vi "CRYFind Insert Locaction in Tree.vi"(6 "sData In":string[](array[string]), 7 "sAction":string, 8 "Index in Step":i32, 9 "Index in Tree":i32, 10 "ParentTag In":string, 11 "Tree in":refnum<vi>) -> (1 "ChildIndex":i32, 2 "ParentTag Out":string, 3 "Tree Out":refnum<vi>)   [LabVIEW 2013]
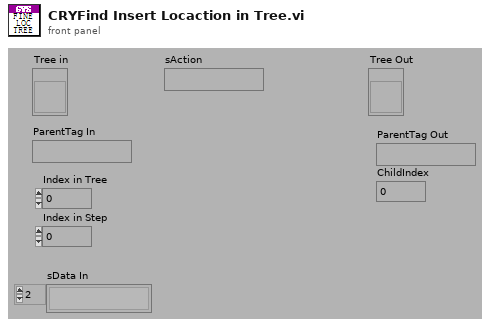
[diagram p1: front panel]
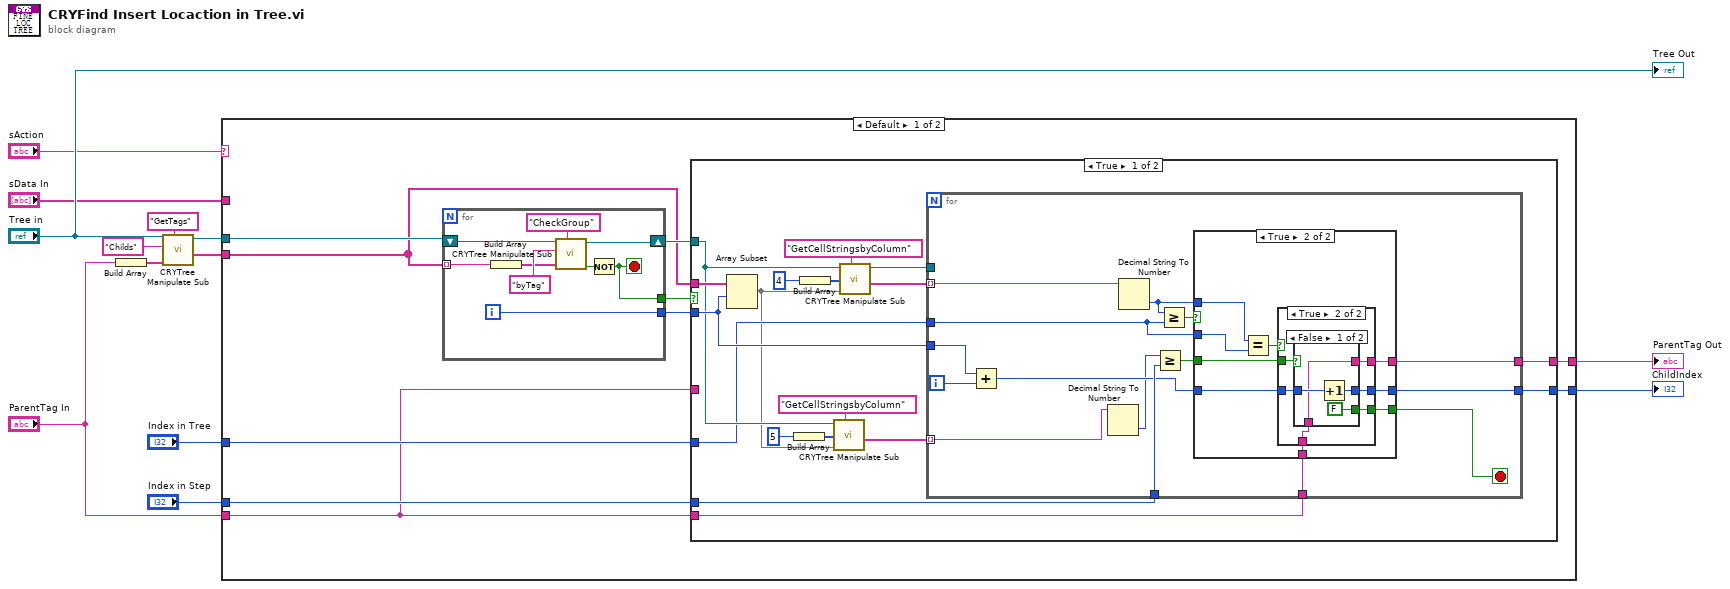
[diagram p0: block diagram]
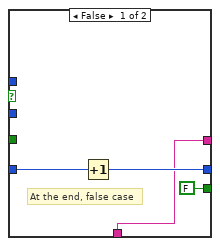
[diagram p2: hidden frame]
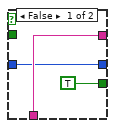
[diagram p3: hidden frame]
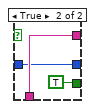
[diagram p4: hidden frame]
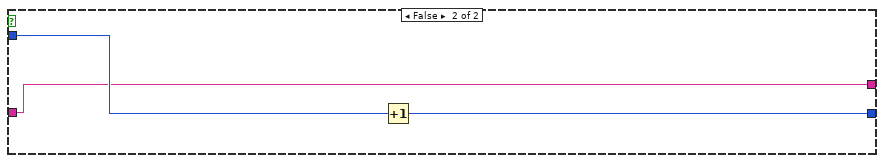
[diagram p5: hidden frame]
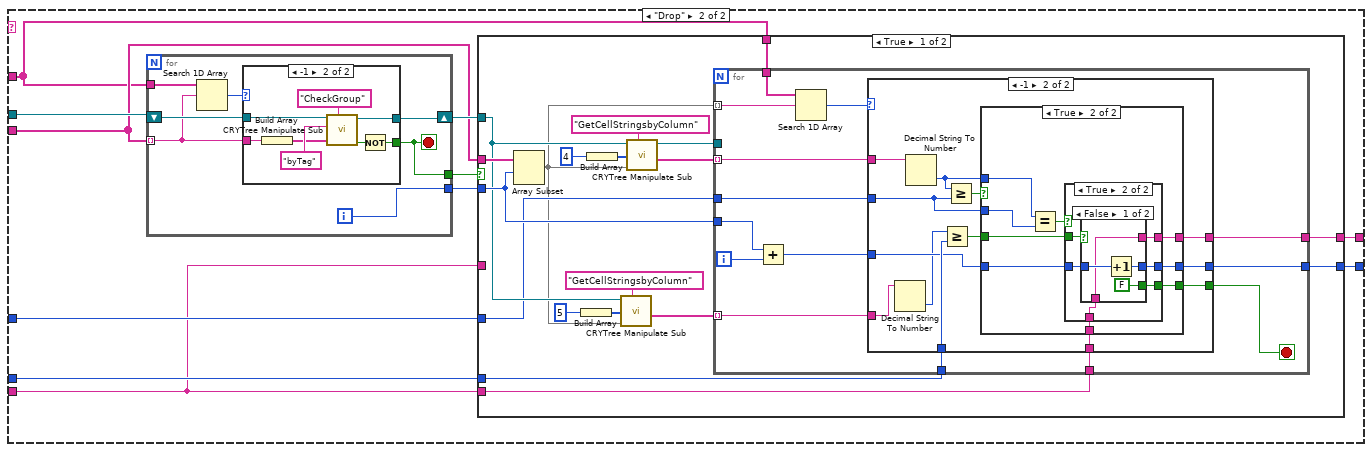
[diagram p6: hidden frame]
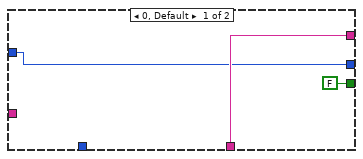
[diagram p7: hidden frame]
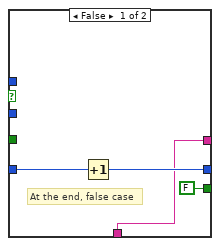
[diagram p8: hidden frame]
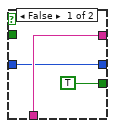
[diagram p9: hidden frame]
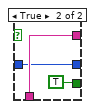
[diagram p10: hidden frame]
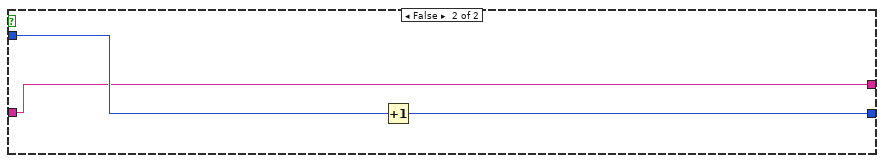
[diagram p11: hidden frame]
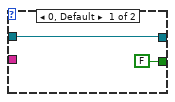
[diagram p12: hidden frame]
diagram:
  n1 = Build Array("ParentTag In") -> (w11:string[])
  n2 = call "CRYTree Manipulate Sub.vi"("sAction"="GetTags", "sData"=w11, "sOption"="Childs", "Tree in"="Tree in") -> ("sData Out"=w3:string[], "Tree Out"=w10:refnum<vi>)  [unwired: 3 in, 3 out]
  n3 = case shown="Default" "sAction" {
    tunnel: w10 -> [w23 w108]
    tunnel: [w19 w104] -> w8
    tunnel: [w18 w103] -> w7
    tunnel: "Index in Tree" -> [w17 w102]
    tunnel: "Index in Step" -> [w16 w101]
    tunnel: "ParentTag In" -> [w15 w100]
    tunnel: w3 -> [w14 w99]
    tunnel: "sData In" -> [_ w98]
    frame Default {
      n4 = for {
        tunnel: w14 -> [w90] mode=indexing
        tunnel: [w95] -> w21
        shift-right: [w91] -> w22
        shift-left: w23 -> [w93]
        tunnel: [w89] -> w20
        i -> [w95]
        stop <- w89 stop-if-true
        n5 = Build Array(w90) -> (w92:string[])
        n6 = call "CRYTree Manipulate Sub.vi"("sAction"="CheckGroup", "sData"=w92, "sOption"="byTag", "Tree in"=w93) -> ("bData out"=w96:bool, "Tree Out"=w91:refnum<vi>)  [unwired: 3 in, 3 out]
        n7 = Not(x=w96) -> (.not. x?=w89:bool)
      }
      n8 = case shown="True" w20 {
        tunnel: w22 -> [w32 _]
        tunnel: [w27 w87] -> w19
        tunnel: [w26 w86] -> w18
        tunnel: w14 -> [w37 _]
        tunnel: w21 -> [w36 w88]
        tunnel: w17 -> [w30 _]
        tunnel: w16 -> [w29 _]
        tunnel: w15 -> [w28 _]
        tunnel: w15 -> [_ w87]
        frame True {
          n9 = Array Subset(array=w37, index=w36) -> (w25:string[])  [unwired: 1 in]
          n10 = Build Array(5 ("nData 2")) -> (w35:i32[])
          n11 = Build Array(4 ("nData 2")) -> (w39:i32[])
          n12 = call "CRYTree Manipulate Sub.vi"("sAction"="GetCellStringsbyColumn", "sData"=w25, "nData"=w35, "Tree in"=w32) -> ("sData Out"=w31:string[])  [unwired: 3 in, 4 out]
          n13 = call "CRYTree Manipulate Sub.vi"("sAction"="GetCellStringsbyColumn", "sData"=w25, "nData"=w39, "Tree in"=w32) -> ("sData Out"=w38:string[], "Tree Out"=w24:refnum<vi>)  [unwired: 3 in, 3 out]
          n14 = for {
            tunnel: w38 -> [w56] mode=indexing
            tunnel: w30 -> [w47]
            tunnel: w36 -> [w54]
            tunnel: w31 -> [w53] mode=indexing
            tunnel: w29 -> [w52]
            tunnel: w28 -> [w51]
            tunnel: [w49] -> w27
            tunnel: [w48] -> w26
            tunnel: w24 -> [_]
            i -> [w55]
            stop <- w46 stop-if-true
            n15 = Add(x=w54, y=w55) -> (x+y=w50:i32)
            n16 = Decimal String To Number(string=w53) -> (number=w45:i32)  [unwired: 2 in, 1 out]
            n17 = Decimal String To Number(string=w56) -> (number=w42:i32)  [unwired: 2 in, 1 out]
            n18 = Greater Or Equal?(x=w45, y=w52) -> (x >= y?=w43:bool)
            n19 = Greater Or Equal?(x=w42, y=w47) -> (x >= y?=w44:bool)
            n20 = case shown="True" w44 {
              tunnel: w51 -> [w57 w68]
              tunnel: w50 -> [w60 w65]
              tunnel: [w57 w67] -> w49
              tunnel: [w58 w66] -> w48
              tunnel: w47 -> [_ w62]
              tunnel: w43 -> [_ w64]
              tunnel: [FALSE w63] -> w46
              tunnel: w42 -> [_ w61]
              frame False {
                # "At the end, false case"
                n21 = Increment(x=w60) -> (x+1=w58:i32)
              }
              frame True {
                n22 = Equal?(x=w61, y=w62) -> (x = y?=w69:bool)
                n23 = case shown="True" w69 {
                  tunnel: w68 -> [w72 w76]
                  tunnel: [w72 w77] -> w67
                  tunnel: [w71 w75] -> w66
                  tunnel: w65 -> [w71 w74]
                  tunnel: w64 -> [_ w78]
                  tunnel: [TRUE w73] -> w63
                  frame False {
                  }
                  frame True {
                    n24 = case shown="False" w78 {
                      tunnel: [w79 w85] -> w77
                      tunnel: w76 -> [w79 w85]
                      tunnel: [w80 w84] -> w75
                      tunnel: w74 -> [w81 w84]
                      tunnel: [FALSE TRUE] -> w73
                      frame False {
                        n25 = Increment(x=w81) -> (x+1=w80:i32)
                      }
                      frame True {
                      }
                    }
                  }
                }
              }
            }
          }
        }
        frame False {
          n26 = Increment(x=w88) -> (x+1=w86:i32)
        }
      }
    }
    frame "Drop" {
      n27 = for {
        tunnel: w99 -> [w190] mode=indexing
        tunnel: [w196] -> w106
        shift-right: [w194] -> w107
        shift-left: w108 -> [w195]
        tunnel: [w193] -> w105
        tunnel: w98 -> [w191]
        i -> [w196]
        stop <- w193 stop-if-true
        n28 = Search 1D Array(1D array=w191, element=w190) -> (index of element=w192:i32)  [unwired: 1 in]
        n29 = case shown="-1" w192 {
          tunnel: w195 -> [w198 w203]
          tunnel: [w198 w201] -> w194
          tunnel: w190 -> [_ w200]
          tunnel: [FALSE w199] -> w193
          frame 0, Default {
          }
          frame -1 {
            n30 = Build Array(w200) -> (w202:string[])
            n31 = call "CRYTree Manipulate Sub.vi"("sAction"="CheckGroup", "sData"=w202, "sOption"="byTag", "Tree in"=w203) -> ("bData out"=w205:bool, "Tree Out"=w201:refnum<vi>)  [unwired: 3 in, 3 out]
            n32 = Not(x=w205) -> (.not. x?=w199:bool)
          }
        }
      }
      n33 = case shown="True" w105 {
        tunnel: w107 -> [w118 _]
        tunnel: [w113 w188] -> w104
        tunnel: [w112 w187] -> w103
        tunnel: w99 -> [w123 _]
        tunnel: w106 -> [w122 w189]
        tunnel: w102 -> [w116 _]
        tunnel: w101 -> [w115 _]
        tunnel: w100 -> [w114 _]
        tunnel: w100 -> [_ w188]
        tunnel: w98 -> [w110 _]
        frame True {
          n34 = Array Subset(array=w123, index=w122) -> (w109:string[])  [unwired: 1 in]
          n35 = Build Array(5 ("nData 2")) -> (w121:i32[])
          n36 = Build Array(4 ("nData 2")) -> (w125:i32[])
          n37 = call "CRYTree Manipulate Sub.vi"("sAction"="GetCellStringsbyColumn", "sData"=w109, "nData"=w121, "Tree in"=w118) -> ("sData Out"=w117:string[])  [unwired: 3 in, 4 out]
          n38 = call "CRYTree Manipulate Sub.vi"("sAction"="GetCellStringsbyColumn", "sData"=w109, "nData"=w125, "Tree in"=w118) -> ("sData Out"=w124:string[], "Tree Out"=w111:refnum<vi>)  [unwired: 3 in, 3 out]
          n39 = for {
            tunnel: w124 -> [w141] mode=indexing
            tunnel: w116 -> [w132]
            tunnel: w122 -> [w139]
            tunnel: w117 -> [w138] mode=indexing
            tunnel: w115 -> [w137]
            tunnel: w114 -> [w136]
            tunnel: [w134] -> w113
            tunnel: [w133] -> w112
            tunnel: w111 -> [_]
            tunnel: w110 -> [w130]
            tunnel: w109 -> [w129] mode=indexing
            i -> [w140]
            stop <- w131 stop-if-true
            n40 = Add(x=w139, y=w140) -> (x+y=w135:i32)
            n41 = Search 1D Array(1D array=w130, element=w129) -> (index of element=w128:i32)  [unwired: 1 in]
            n42 = case shown="-1" w128 {
              tunnel: w141 -> [_ w157]
              tunnel: w138 -> [_ w156]
              tunnel: w137 -> [_ w155]
              tunnel: w136 -> [w143 w154]
              tunnel: w135 -> [w142 w153]
              tunnel: [w143 w152] -> w134
              tunnel: [w142 w151] -> w133
              tunnel: w132 -> [_ w150]
              tunnel: [FALSE w149] -> w131
              frame 0, Default {
              }
              frame -1 {
                n43 = Decimal String To Number(string=w156) -> (number=w148:i32)  [unwired: 2 in, 1 out]
                n44 = Decimal String To Number(string=w157) -> (number=w145:i32)  [unwired: 2 in, 1 out]
                n45 = Greater Or Equal?(x=w148, y=w155) -> (x >= y?=w146:bool)
                n46 = Greater Or Equal?(x=w145, y=w150) -> (x >= y?=w147:bool)
                n47 = case shown="True" w147 {
                  tunnel: w154 -> [w158 w169]
                  tunnel: w153 -> [w161 w166]
                  tunnel: [w158 w168] -> w152
                  tunnel: [w159 w167] -> w151
                  tunnel: w150 -> [_ w163]
                  tunnel: w146 -> [_ w165]
                  tunnel: [FALSE w164] -> w149
                  tunnel: w145 -> [_ w162]
                  frame False {
                    # "At the end, false case"
                    n48 = Increment(x=w161) -> (x+1=w159:i32)
                  }
                  frame True {
                    n49 = Equal?(x=w162, y=w163) -> (x = y?=w170:bool)
                    n50 = case shown="True" w170 {
                      tunnel: w169 -> [w173 w177]
                      tunnel: [w173 w178] -> w168
                      tunnel: [w172 w176] -> w167
                      tunnel: w166 -> [w172 w175]
                      tunnel: w165 -> [_ w179]
                      tunnel: [TRUE w174] -> w164
                      frame False {
                      }
                      frame True {
                        n51 = case shown="False" w179 {
                          tunnel: [w180 w186] -> w178
                          tunnel: w177 -> [w180 w186]
                          tunnel: [w181 w185] -> w176
                          tunnel: w175 -> [w182 w185]
                          tunnel: [FALSE TRUE] -> w174
                          frame False {
                            n52 = Increment(x=w182) -> (x+1=w181:i32)
                          }
                          frame True {
                          }
                        }
                      }
                    }
                  }
                }
              }
            }
          }
        }
        frame False {
          n53 = Increment(x=w189) -> (x+1=w187:i32)
        }
      }
    }
  }
  "ParentTag Out" <- w8
  "ChildIndex" <- w7
  "Tree Out" <- "Tree in"
